vi "dlqr.vi"(9 "Input Weight":T1, 10 "Process Weight":T1, 11 "Plant":T2={"Gains"={"A"=[[0.0, 1.0], [0.0, -166.98]], "B"=[[0.0], [16.43]], "C"=[[1.0, 0.0]], "D"=[[0.0]], "Q"=[[0.005, 0.0], [0.0, 0.005]], "R"=[[0.005]], "K"=[[24.345709068776628, -7.72854534388314]], "Kff"=[[0.0, 10.536652546185671]], "L"=[[0.618], [0.0]]}, "X"=[[0.0], [0.0]]}) -> (3 "Plant Out":T2={"Gains"={"A"=[[0.0, 1.0], [0.0, -166.98]], "B"=[[0.0], [16.43]], "C"=[[1.0, 0.0]], "D"=[[0.0]], "Q"=[[0.005, 0.0], [0.0, 0.005]], "R"=[[0.005]], "K"=[[24.345709068776628, -7.72854534388314]], "Kff"=[[0.0, 10.536652546185671]], "L"=[[0.618], [0.0]]}, "X"=[[0.0], [0.0]]})   [LabVIEW 2017]
uses:
  <vilib>/Analysis/Matrix/Datatypes/RealMatrix.ctl
  <vilib>/Analysis/Matrix/Numeric/Conversions/Array To Matrix - RA2.vi
  <vilib>/Analysis/Matrix/NI_Matrix.lvlib
panel:
  out "standard output":string
  out "standard error":string
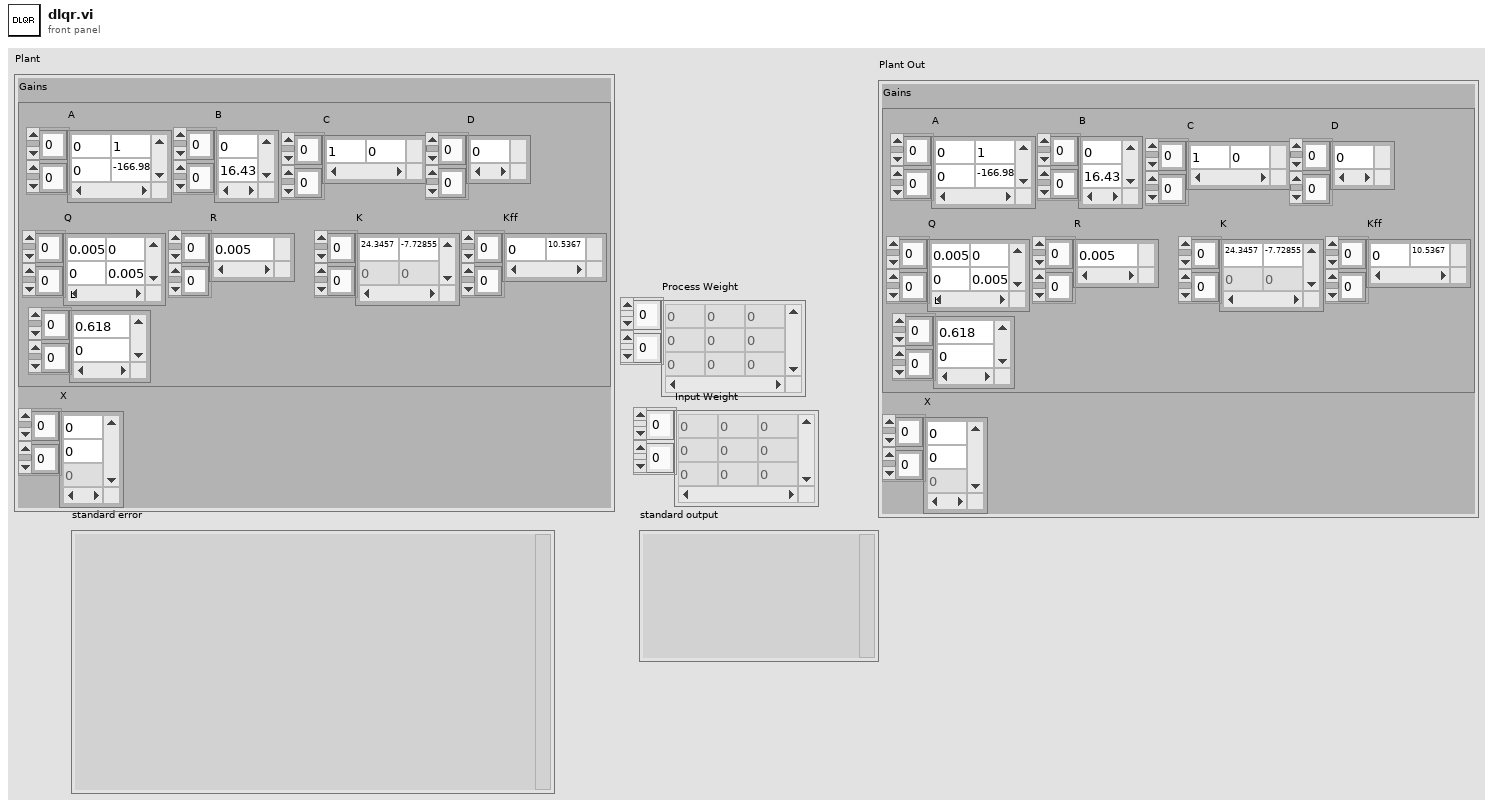
[diagram p1: front panel]
types:
  T1 = typedef "NI_Matrix.lvlib/RealMatrix.ctl" = dbl[][]
  T2 = cluster{"Gains":cluster{"A":T1, "B":T1, "C":T1, "D":T1, "Q":T1, "R":T1, "K":T1, "Kff":T1, "L":T1}, "X":T1}
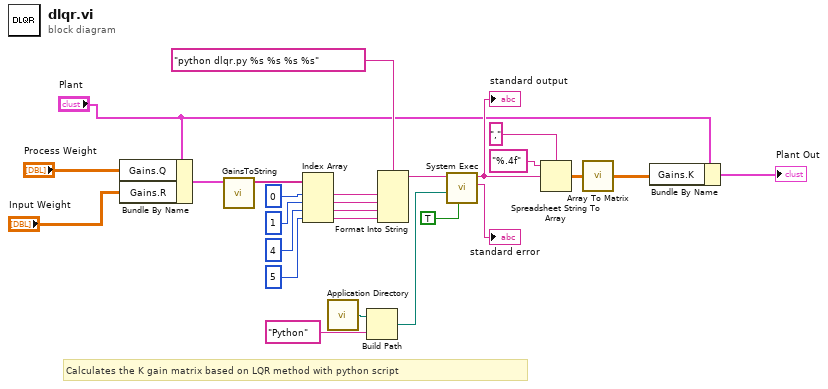
[diagram p0: block diagram]
diagram:
  # "Calculates the K gain matrix based on LQR method with python script"
  n1 = Bundle By Name(cluster="Plant", "Gains.Q"="Process Weight", "Gains.R"="Input Weight") -> (w6:T2)
  n2 = call "GainsToString.vi"("Plant"=w6) -> ("Strings"=w19:string[])  [unwired: 10 in]
  n3 = Index Array(array=w19, index #1=0 ("index"), index #2=1 ("index"), index #3=4 ("index"), index #4=5 ("index")) -> (element #1=w18:string, element #2=w17:string, element #3=w14:string, element #4=w13:string)
  n4 = call <vilib>:"Application Directory.vi"() -> ("Application Directory"=w26:path)
  n5 = Build Path(base path=w26, name or relative path="Python") -> (appended path=w24:path)
  n6 = Format Into String(format string="python dlqr.py %s %s %s %s" ("command line"), w18, w17, w14, w13) -> (resulting string=w20:string)  [unwired: 2 in, 1 out]
  n7 = call <vilib>:"System Exec.vi"("run minimized? (F)"=TRUE, "working directory"=w24, "command line"=w20) -> ("standard error"=→"standard error":string, "standard output"=w8:string)  [unwired: 5 in, 2 out]
  "standard output" <- w8
  n8 = Spreadsheet String To Array(delimiter (Tab)=",", format string="%.4f", spreadsheet string=w8) -> (array=w7:dbl[][])  [unwired: 1 in]
  n9 = call-poly <vilib>:"Array To Matrix.vi"("Real 2D Array"=w7) -> ("Real Matrix"=w3:T1)
  n10 = Bundle By Name(cluster="Plant", "Gains.K"=w3) -> (→"Plant Out":T2)
